vi "E12_Form_Node.vi"() -> ()   [LabVIEW 2020]
panel:
  out "X2":cdb
  out "X1":cdb
  in  "c":dbl
  in  "b":dbl
  in  "a":dbl
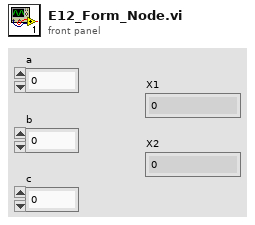
[diagram p1: front panel]
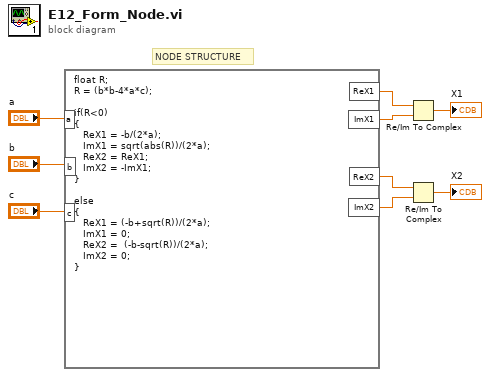
[diagram p0: block diagram]
diagram:
  # "NODE STRUCTURE"
  n1 = formula code="float R;\nR = (b*b-4*a*c);\n\nif(R<0)\n{\n   ReX1 = -b/(2*a);\n   ImX1 = sqrt(abs(R))/(2*a);\n   ReX2 = ReX1;\n   ImX2 = -ImX1;\n}\n\nelse\n{\n   ReX1 = (-b+sqrt(R))/(2*a);\n   ImX1 = 0;\n   ReX2 =  (-b-sqrt(R))/(2*a);\n   ImX2 = 0;\n}"("a"="a", "b"="b", "c"="c") -> ("ImX2"=w3:dbl, "ReX1"=w6:dbl, "ImX1"=w5:dbl, "ReX2"=w4:dbl)
  n2 = Re/Im To Complex(1:w5, 2:w6) -> (0:→"X1":cdb)
  n3 = Re/Im To Complex(1:w3, 2:w4) -> (0:→"X2":cdb)
